vi "Getpower.vi"(1 "Wavlength array":dbl[](array[numeric])=[400.0, 425.0, 450.0, 475.0, 500.0], 2 "Normalizing power wave":dbl[][](array[numeric])=[[1.0, 400.0], [2.0, 450.0], [1.0, 500.0]]) -> (0 "Power array out":dbl[](array[numeric])=[1.0, 1.5, 2.0, 1.5, 1.0])   [LabVIEW 2013]
panel:
  out "Fractional index":dbl=2.0
  out "closest index":i32=2
  out "closest element":dbl=500.0
  in  "start index (0)":i32
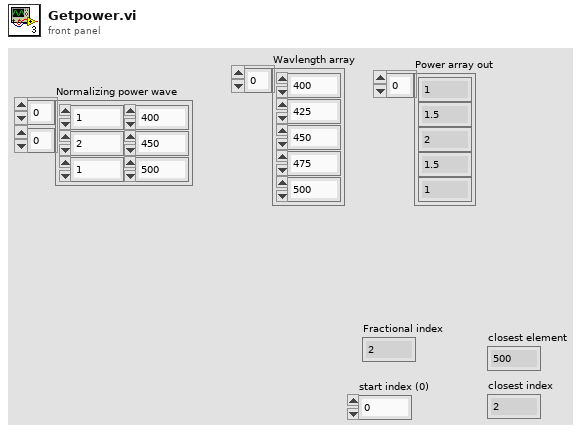
[diagram p1: front panel]
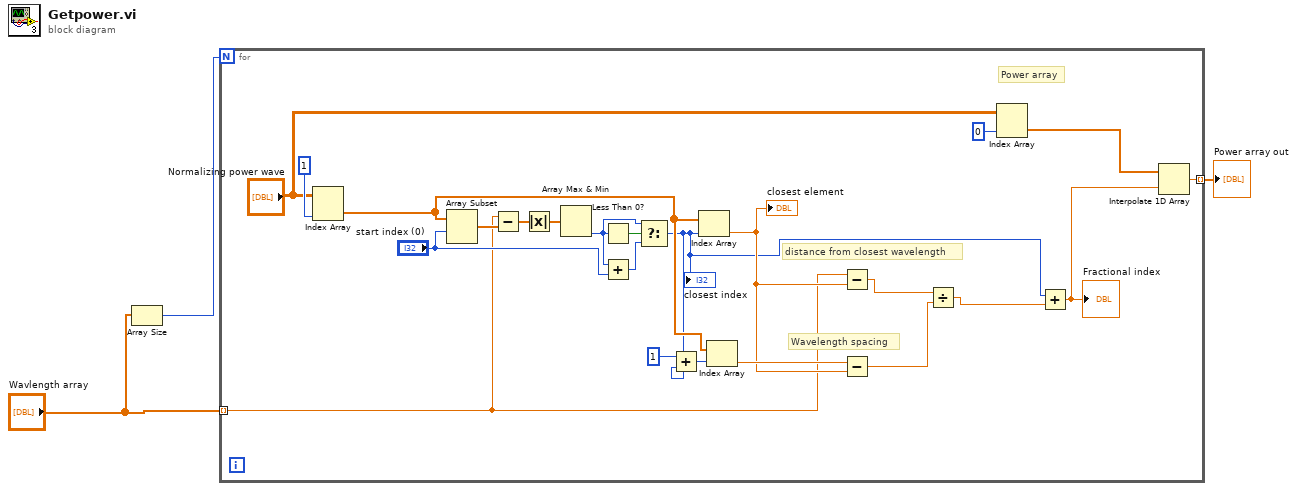
[diagram p0: block diagram]
diagram:
  n1 = Array Size(array="Wavlength array") -> (size(s)=w1:i32)
  n2 = for {
    N: w1 -> [_]
    tunnel: [w5] -> w3 mode=indexing
    tunnel: "Wavlength array" -> [w4] mode=indexing
    # "Power array"
    # "distance from closest wavelength"
    # "Wavelength spacing"
    n3 = Index Array(array="Normalizing power wave", index (col)=1 ("disabled index (col)")) -> (element=w14:dbl[])  [unwired: 1 in]
    n4 = Array Subset(array=w14, index="start index (0)") -> (w26:dbl[])  [unwired: 1 in]
    n5 = Subtract(x=w4, y=w26) -> (x-y=w20:dbl[])
    n6 = Absolute Value(x=w20) -> (abs(x)=w22:dbl[])
    n7 = Array Max & Min(array=w22) -> (min index (indices)=w24:i32)  [unwired: 3 out]
    n8 = Less Than 0?(x=w24) -> (x < 0?=w23:bool)
    n9 = Add(x=w24, y="start index (0)") -> (x+y=w25:i32)
    n10 = Select(t=w24, s=w23, f=w25) -> (s? t:f=w9:i32)
    "closest index" <- w9
    n11 = Add(x=1, y=w9) -> (x+y=w15:i32)
    n12 = Index Array(array=w14, index=w9) -> (element=w12:dbl)
    "closest element" <- w12
    n13 = Index Array(array=w14, index=w15) -> (element=w13:dbl)
    n14 = Subtract(x=w4, y=w12) -> (x-y=w11:dbl)
    n15 = Subtract(x=w13, y=w12) -> (x-y=w10:dbl)
    n16 = Divide(x=w11, y=w10) -> (x/y=w8:dbl)
    n17 = Index Array(array="Normalizing power wave", index (col)=0) -> (element=w7:dbl[])  [unwired: 1 in]
    n18 = Add(x=w9, y=w8) -> (x+y=w6:dbl)
    "Fractional index" <- w6
    n19 = Interpolate 1D Array(1:w6, 2:w7) -> (0:w5:dbl)
  }
  "Power array out" <- w3
